vi "Move and Hide All.vi"(0 "Cluster Refs":refnum<vi>[](array[refnum]), 2 "Visible":bool, 11 "Sub Panel Refs":refnum<vi>[](array[refnum])) -> (4 "Cluster Refs Dup":refnum<vi>[](array[refnum]), 15 "Sub Panel Refs Dup":refnum<vi>[](array[refnum]))   [LabVIEW 2016]
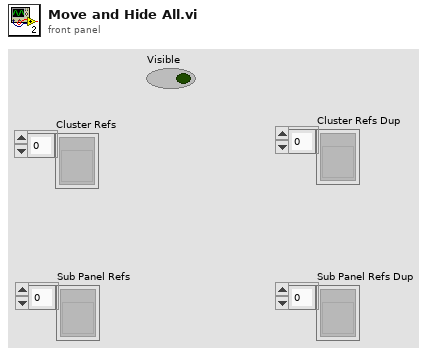
[diagram p1: front panel]
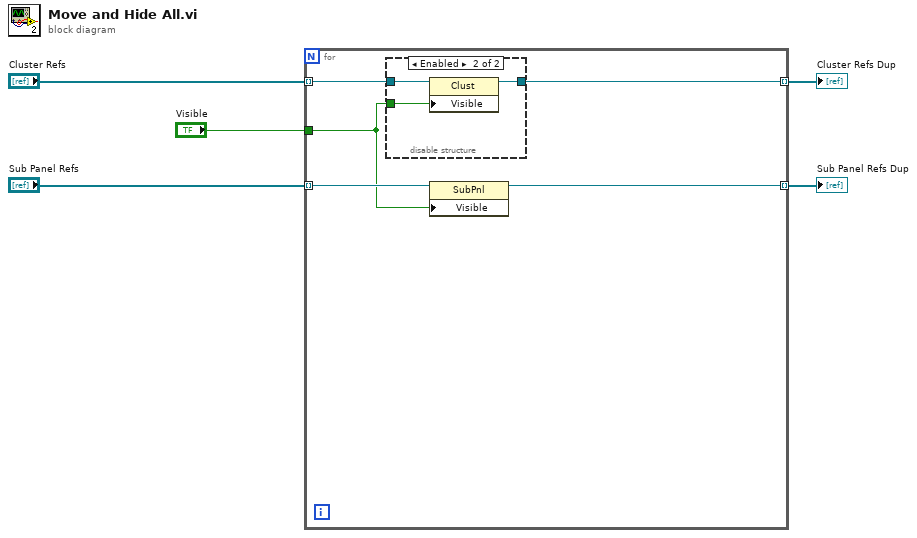
[diagram p0: block diagram]
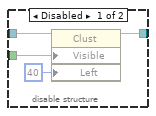
[diagram p2: hidden frame]
diagram:
  n1 = for {
    tunnel: "Cluster Refs" -> [w10] mode=indexing
    tunnel: "Sub Panel Refs" -> [w9] mode=indexing
    tunnel: [w8] -> w3 mode=indexing
    tunnel: [w7] -> w2 mode=indexing
    tunnel: "Visible" -> [w6]
    n2 = disable-structure shown="Enabled" {
      disable-tunnel: w10 -> [w14 w17]
      disable-tunnel: [w13 w16] -> w8
      disable-tunnel: w6 -> [w12 w15]
      frame Disabled {
        n3 = property class="Clust"(reference=w14, "Visible"=w12, "Left"=40 ("Position:Left")) -> (reference out=w13:refnum<vi>)  [unwired: 1 in, 1 out]
      }
      frame Enabled {
        n4 = property class="Clust"(reference=w17, "Visible"=w15) -> (reference out=w16:refnum<vi>)  [unwired: 1 in, 1 out]
      }
    }
    n5 = property class="SubPnl"(reference=w9, "Visible"=w6) -> (reference out=w7:refnum<vi>)  [unwired: 1 in, 1 out]
  }
  "Cluster Refs Dup" <- w3
  "Sub Panel Refs Dup" <- w2
